vi "SetCoupling.vi"(0 "reference in":refnum<class "Frequency_Counter_TTi.lvclass">, 5 "error in (no error)":errorcluster) -> (14 "reference in":refnum<class "Frequency_Counter_TTi.lvclass">, 19 "error out":errorcluster)   [LabVIEW 2022 SP3, in "Frequency_Counter_TTi.lvlib" / "Frequency_Counter_TTi.lvclass"]
uses:
  Frequency_Counter_TTi.lvclass
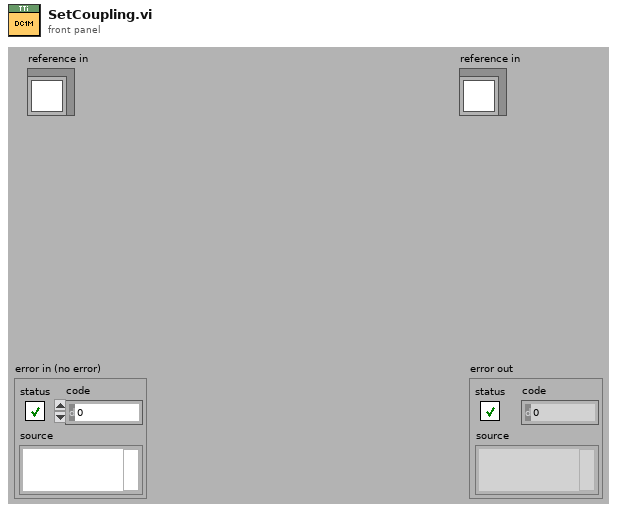
[diagram p1: front panel]
types:
  T1 = typedef "Frequency_Counter_TTi.lvlib/Frequency_Counter_TTi.lvclass/ObjectAttributes.ctl" = cluster{"Config":T2, "Freq":dbl}
  T2 = typedef "Frequency_Counter_TTi.lvlib/Frequency_Counter_TTi.lvclass/Config.ctl" = cluster{"ComPort":refnum<visa-resource-name>}
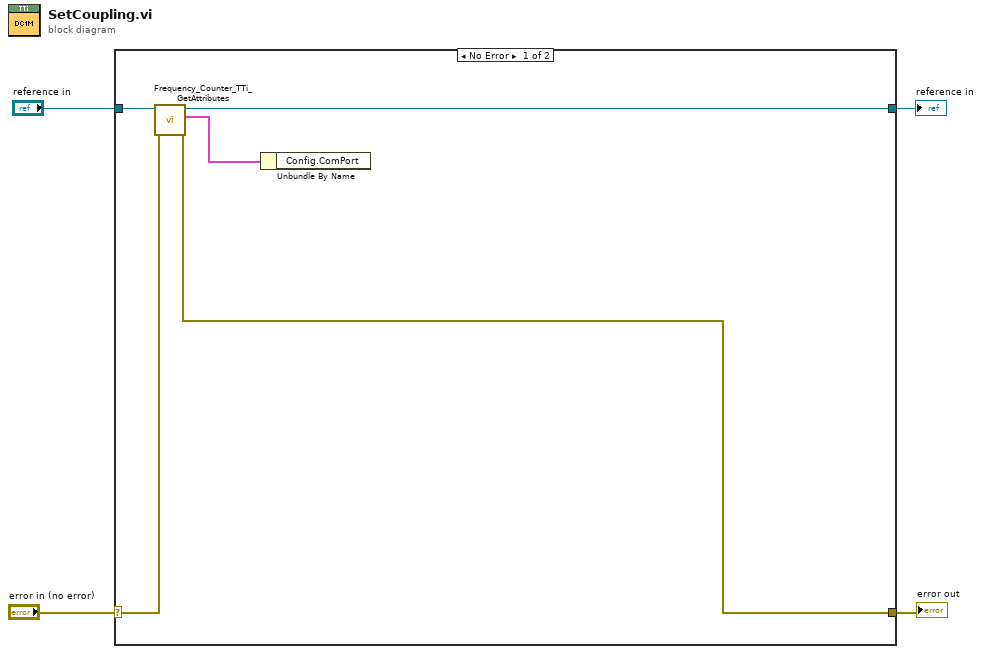
[diagram p0: block diagram]
diagram:
  n1 = case shown="No Error" "error in (no error)" {
    selector: "error in (no error)" -> [w9 w11]
    tunnel: [w5 w11] -> w3
    tunnel: [w6 w10] -> w1
    tunnel: "reference in" -> [w7 w10]
    frame No Error {
      n2 = call "Frequency_Counter_TTi_GetAttributes.vi"("error in (no error)"=w9, "reference in"=w7) -> ("error out"=w5:errorcluster, "Data"=w8:T1, "reference out"=w6:refnum<class "Frequency_Counter_TTi.lvclass">)  [unwired: 6 in, 1 out]
      n3 = Unbundle By Name(w8) -> ()  [unwired: 1 out]
    }
    frame Error {
    }
  }
  "error out" <- w3
  "reference in" <- w1
